vi "Main_03B.vi"() -> ()   [LabVIEW 2025]
uses:
  Utility/Universal Utility/TypeDefs_Utility/Cluster_Row-Column.ctl
  9e3f57c0-2ef8-4495-8287-c6a42a5fb955.vi
  Utility/Universal Utility/TypeDefs_Utility/ENUM_4 Directions U-D-L-R.ctl
  Utility/Universal Utility/TypeDefs_Utility/ENUM_8 Directions U-D-L-R.ctl
panel:
  out "number":u64
  out "Joltage LIst":u64[](array[numeric])
  out "MATCH":bool
  in  "Select Data":enum32{"Example", "Puzzle"}(tab)
  in  "EX Target":u64=357
  in  "Example":string="987654321111111\n811111111111119\n234234234234278\n818181911112111"
  in  "Puzzle":string="2233643232222242333443433223122333324326451323323334325223136631334332233233323164354342233332238233\n6436547659356357277564683346658554864789866767856546426667566576537557576764753366663247799566575359\n4322212422212222222222112222221252322222222222121152214312222222226122122421262632221222352222223522\n5242873574376258254526262841222235756126125363535226724625252231422222223232432416114933476433226425\n4423241233122222212222152223222321224343432221222131223143222222223442622361254132221212223321223232\n23544433354444444444454732334364434434474343434534643724444447444443414354445434434336456444466..."
  in  "Puzzle Target":u64=169512729575727
  out "Answer":u64
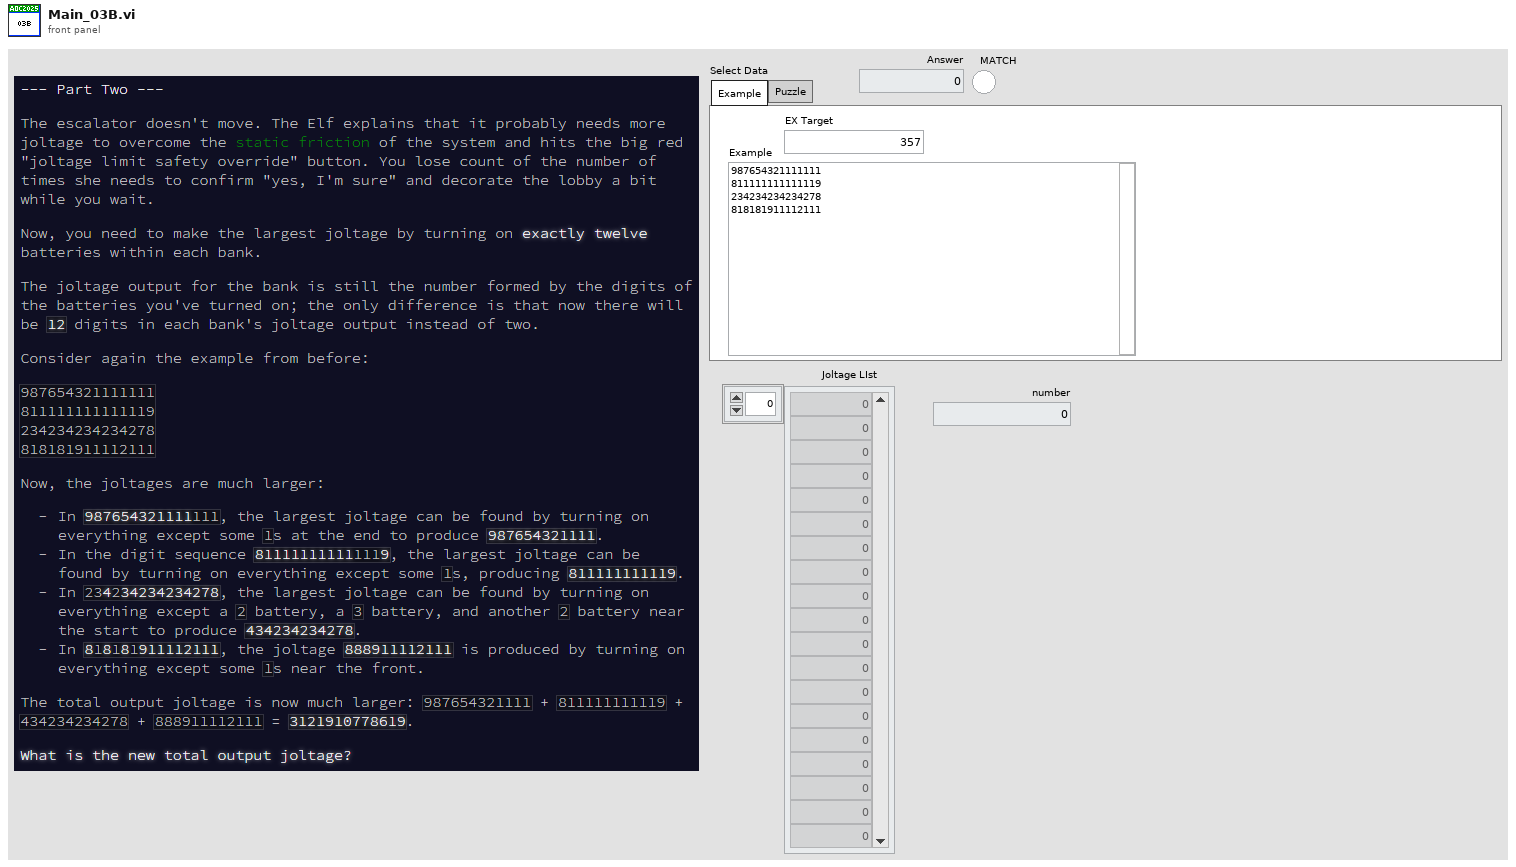
[diagram p1: front panel]
types:
  T1 = typedef "ENUM_8 Directions U-D-L-R.ctl" = enum16{"Up;-1,0", "Up-Right;-1,1", "Right;0,1", "Down-Right;1,1", "Down;1,0", "Down-Left;1,-1", "Left;0,-1", "Up-Left;-1,-1"}
  T2 = typedef "ENUM_4 Directions U-D-L-R.ctl" = enum16{"Up;-1,0", "Right;0,1", "Down;1,0", "Left;0,-1"}
  T3 = typedef "Cluster_Row-Column.ctl" = cluster{"R":i32, "C":i32}
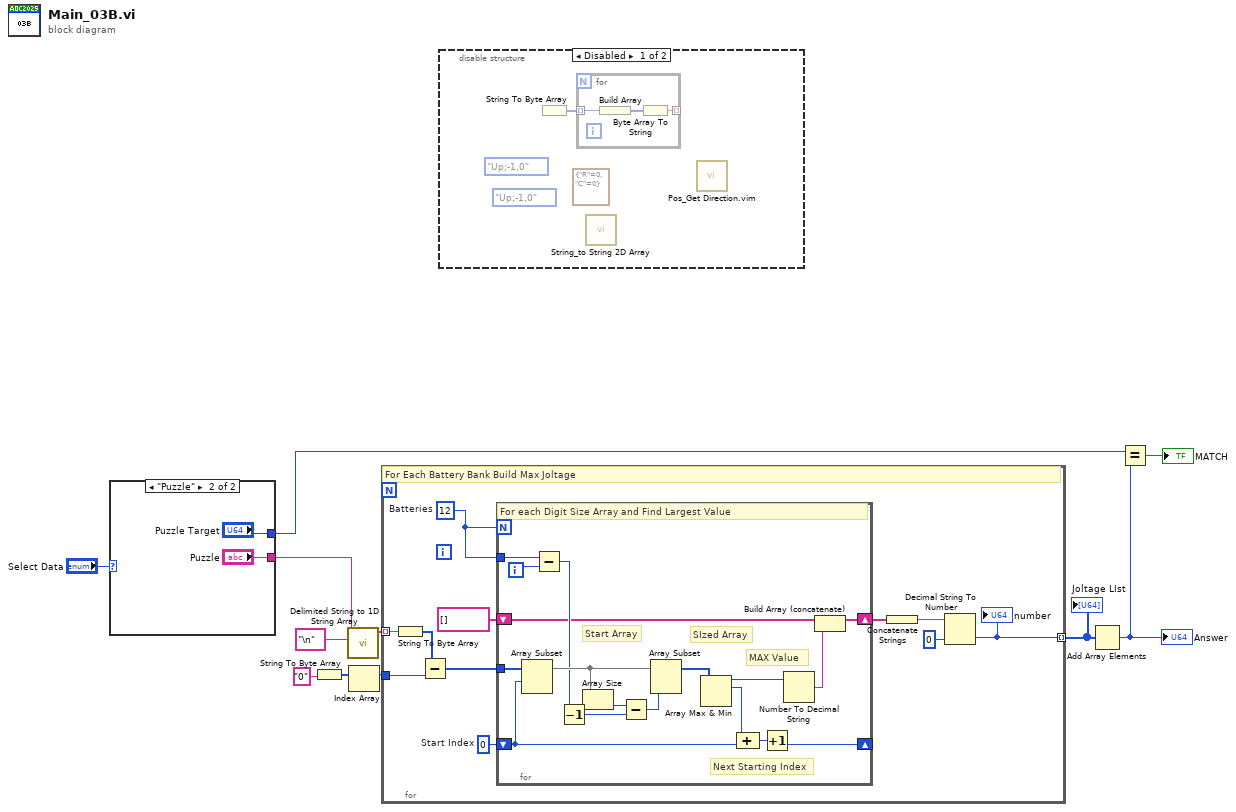
[diagram p0: block diagram]
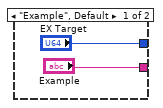
[diagram p2: hidden frame]
diagram:
  n1 = case shown="\"Puzzle\"" "Select Data" {
    tunnel: ["Example" "Puzzle"] -> w9
    tunnel: ["EX Target" "Puzzle Target"] -> w6
    frame "Example", Default {
    }
    frame "Puzzle" {
    }
  }
  n2 = String To Byte Array(string="0") -> (unsigned byte array=w5:u8[])
  n3 = call <vilib>:"Delimited String to 1D String Array.vi"("delimiter"="\n" ("delimiter (Tab)"), "delimited string"=w9) -> ("string array"=w10:string[])  [unwired: 9 in]
  n4 = Index Array(array=w5) -> (element=w3:u8)  [unwired: 1 in]
  n5 = for {
    tunnel: w10 -> [w25] mode=indexing
    tunnel: w3 -> [w22]
    tunnel: [w16] -> w2 mode=indexing
    w20 = 0  # Start Index
    w19 = 12  # Batteries
    # "For Each Battery Bank Build Max Joltage"
    n6 = String To Byte Array(string=w25) -> (unsigned byte array=w26:u8[])
    n7 = Subtract(x=w26, y=w22) -> (x-y=w24:u8[])
    n8 = for {
      N: w19 -> [_]
      tunnel: w24 -> [w39]
      shift-right: [w30] -> _
      shift-left: w20 -> [w28]
      shift-right: [w32] -> w23
      shift-left: string[] [] -> [w33]
      tunnel: w19 -> [w36]
      i -> [w35]
      # "Next Starting Index"
      # "MAX Value"
      # "SIzed Array"
      # "Start Array"
      # "For each Digit Size Array and Find Largest Value"
      n9 = Array Subset(array=w39, index=w28) -> (w38:u8[])  [unwired: 1 in]
      n10 = Subtract(x=w36, y=w35) -> (x-y=w34:i32)
      n11 = Decrement(x=w34) -> (x-1=w37:i32)
      n12 = Array Size(array=w38) -> (size(s)=w40:i32)
      n13 = Subtract(x=w40, y=w37) -> (x-y=w41:i32)
      n14 = Array Subset(array=w38, length=w41) -> (w43:u8[])  [unwired: 1 in]
      n15 = Array Max & Min(array=w43) -> (max value=w31:u8, max index (indices)=w42:i32)  [unwired: 2 out]
      n16 = Compound Arithmetic op=ADD(w42, w28) -> (w29:i32)
      n17 = Increment(x=w29) -> (x+1=w30:i32)
      n18 = Number To Decimal String(number=w31) -> (decimal integer string=w27:string)  [unwired: 1 in]
      n19 = Build Array (concatenate)(w33, w27) -> (w32:string[])
    }
    n20 = Concatenate Strings(w23) -> (w18:string)
    n21 = Decimal String To Number(string=w18, default (0L)=u64 0 ("default (0 I32)")) -> (number=w16:u64)  [unwired: 1 in, 1 out]
    "number" <- w16
  }
  "Joltage LIst" <- w2
  n22 = disable-structure shown="Disabled" {
    frame Disabled {
      (unwired) ENUM_8_Directions_U-D-L-R."Up;-1,0" ("Direction 8")
      (unwired) ENUM_4_Directions_U-D-L-R."Up;-1,0" ("Direction")
      (unwired) T3 {"R"=0, "C"=0} ("Position")
      n23 = String To Byte Array() -> (unsigned byte array=w44:u8[])  [unwired: 1 in]
      n24 = for {
        tunnel: w44 -> [w47] mode=indexing
        tunnel: [w45] -> _ mode=indexing
        n25 = Build Array(w47) -> (w46:u8[])
        n26 = Byte Array To String(unsigned byte array=w46) -> (string=w45:string)
      }
      n27 = call "String_to String 2D Array.vi"() -> ()  [unwired: 11 in, 1 out]
      n28 = call "Pos_Get Direction.vim"() -> ()  [unwired: 11 in, 1 out]
    }
    frame Enabled {
    }
  }
  n29 = Add Array Elements(numeric array=w2) -> (sum=w1:u64)
  "Answer" <- w1
  n30 = Equal?(x=w6, y=w1) -> (x = y?=→"MATCH":bool)
